vi "Sensor_Color.vi"(0 "COM Bluegiga in":refnum<visa-resource-name>, 3 "error in (no error)":errorcluster) -> (7 "COM Bluegiga out":refnum<visa-resource-name>, 8 "subarray":u8[](array[numeric]), 9 "Color":u32(colorbox), 10 "error out":errorcluster)   [LabVIEW 2020]
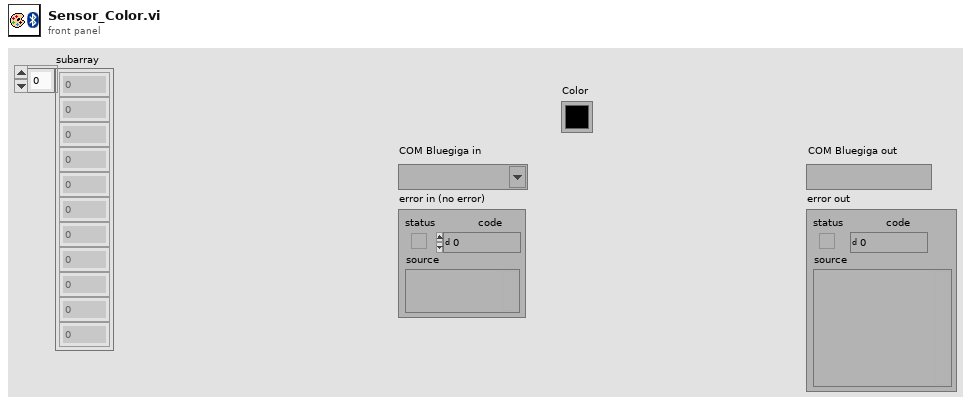
[diagram p1: front panel]
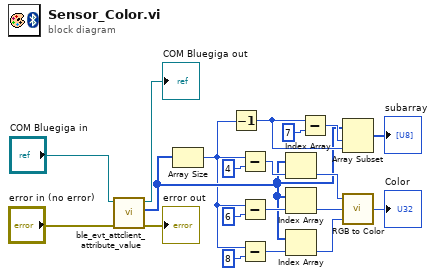
[diagram p0: block diagram]
diagram:
  n1 = call <vilib>:"ble_evt_attclient_attribute_value.vi"("error in (no error)"="error in (no error)", "COM Bluegiga in"="COM Bluegiga in") -> ("error out"=→"error out":errorcluster, "characteristic value"=w3:u8[], "COM Bluegiga out"=→"COM Bluegiga out":refnum<visa-resource-name>)  [unwired: 6 in, 1 out]
  n2 = Array Size(array=w3) -> (size(s)=w2:i32)
  n3 = Decrement(x=w2) -> (x-1=w14:i32)
  n4 = Subtract(x=w2, y=4) -> (x-y=w11:i32)
  n5 = Subtract(x=w2, y=6) -> (x-y=w9:i32)
  n6 = Subtract(x=w2, y=8) -> (x-y=w7:i32)
  n7 = Index Array(array=w3, index=w11) -> (element=w12:u8)
  n8 = Index Array(array=w3, index=w9) -> (element=w5:u8)
  n9 = Index Array(array=w3, index=w7) -> (element=w4:u8)
  n10 = Subtract(x=w14, y=7 ("x")) -> (x-y=w15:i32)
  n11 = Array Subset(array=w3, index=w15, length=w14) -> (→"subarray":u8[])
  n12 = call <vilib>:"RGB to Color.vi"("B"=w4, "G"=w5, "R"=w12) -> ("Color"=→"Color":u32)
